vi "set password protection on all VIs.vi"() -> ()   [LabVIEW 2012]
panel:
  in  "keep GFG unlocked":bool
  out "File Path":path
  in  "Confirm New Password":string="password"
  in  "Ring":u16(ring)=2 items=["Unlock", "set new password", "change password"]
  in  "New Password":string="password"
  in  "Old Password":string="password"
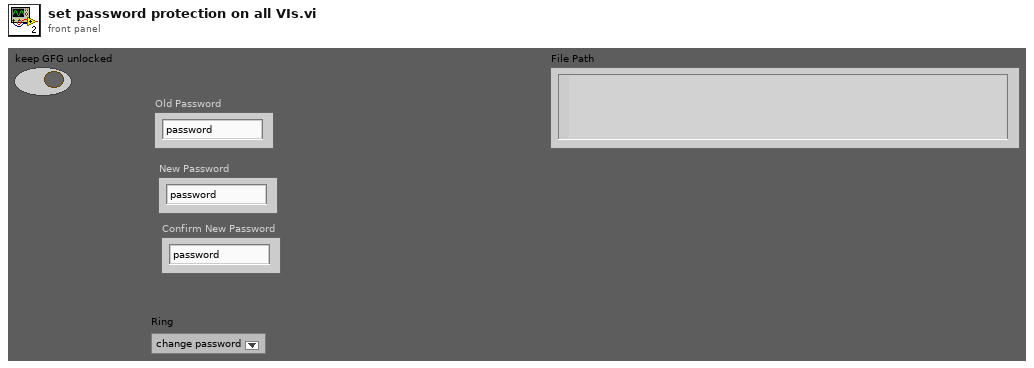
[diagram p1: front panel]
types:
  T1 = enum32{"invalid lock state", "Not Locked", "Locked (No Password)", "Password-protected"}
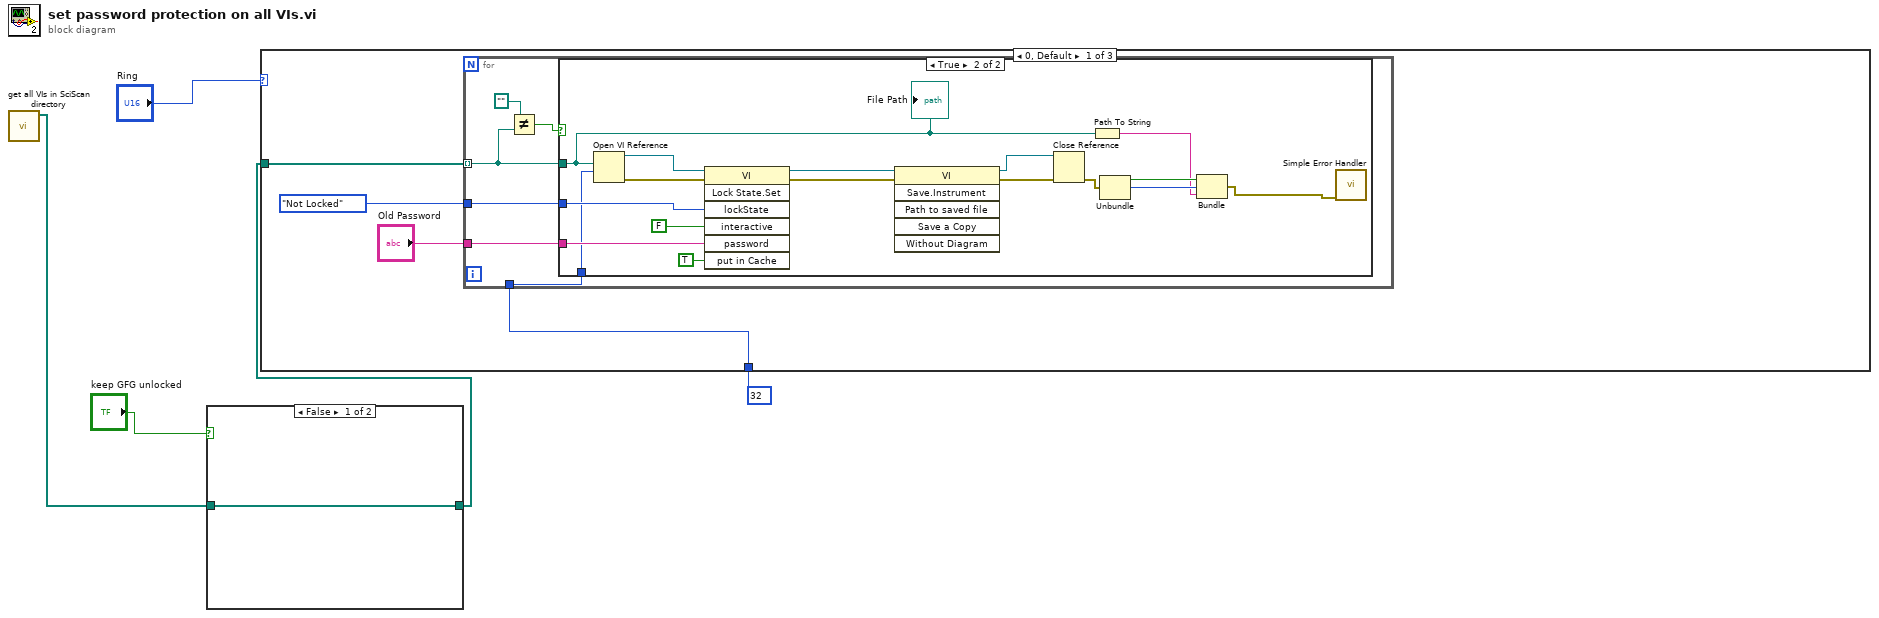
[diagram p0: block diagram]
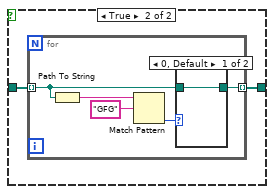
[diagram p2: hidden frame]
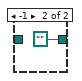
[diagram p3: hidden frame]
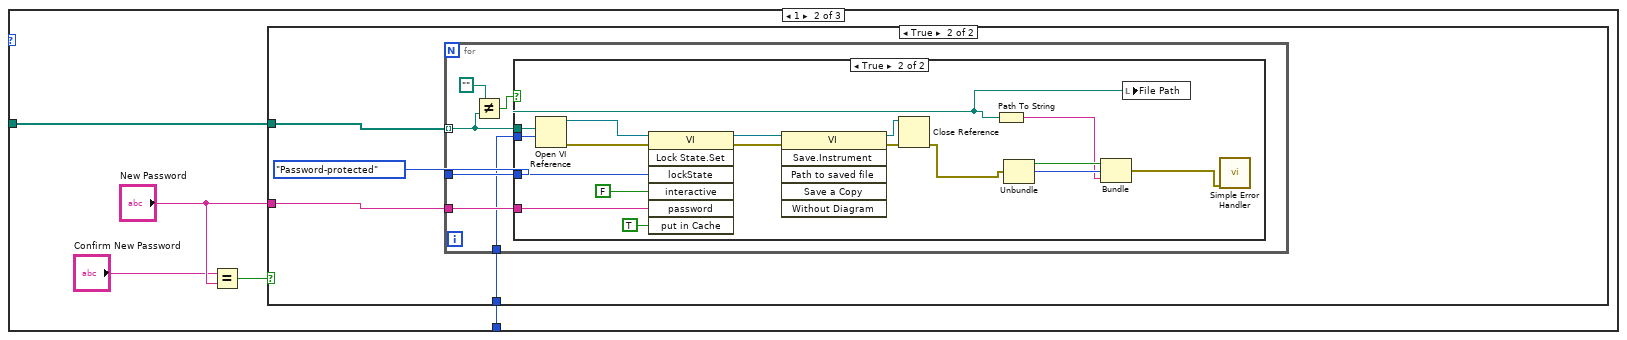
[diagram p5: hidden frame]
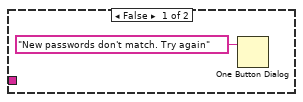
[diagram p6: hidden frame]
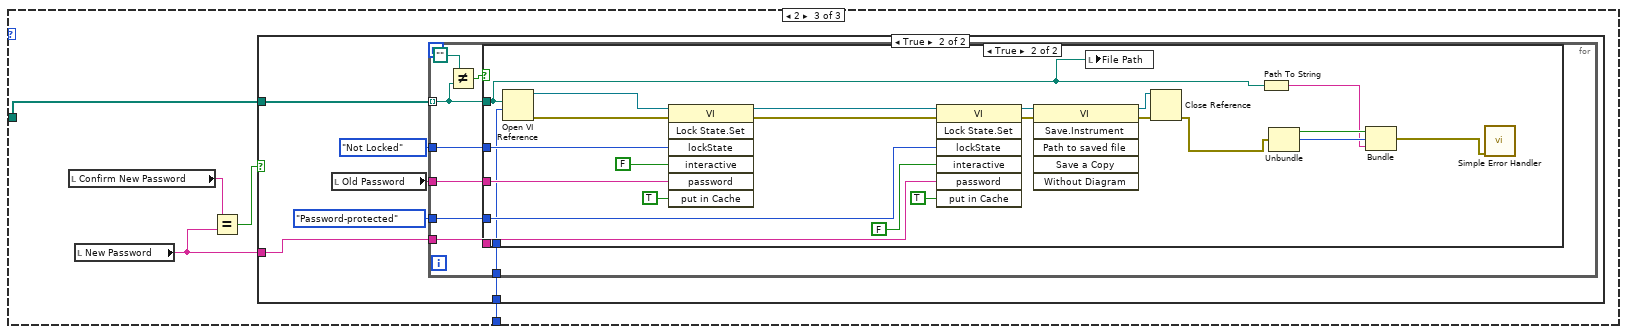
[diagram p8: hidden frame]
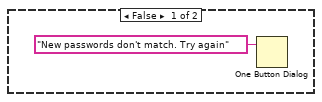
[diagram p9: hidden frame]
diagram:
  n1 = call "get all VIs in SciScan directory.vi"() -> ("All Files in Dir"=w2:path[])  [unwired: 11 in]
  n2 = case shown="False" "keep GFG unlocked" {
    tunnel: [w6 w8] -> w1
    tunnel: w2 -> [w6 w7]
    frame False {
    }
    frame True {
      n3 = for {
        tunnel: [w10] -> w8 mode=indexing
        tunnel: w7 -> [w9] mode=indexing
        n4 = Path To String(path=w9) -> (string=w13:string)
        n5 = Match Pattern(string=w13, regular expression="GFG") -> (offset past match=w11:i32)  [unwired: 1 in, 3 out]
        n6 = case shown="0, Default" w11 {
          tunnel: [w14 path ""] -> w10
          tunnel: w9 -> [w14 _]
          frame 0, Default {
          }
          frame -1 {
          }
        }
      }
    }
  }
  n7 = case shown="0, Default" "Ring" {
    tunnel: w1 -> [w19 w47 w80]
    tunnel: 32 ("options") -> [w16 w43 w76]
    frame 0, Default {
      n8 = for {
        tunnel: w19 -> [w21] mode=indexing
        tunnel: "Old Password" -> [w25]
        tunnel: T1."Not Locked" ("Lock State") -> [w24]
        tunnel: w16 -> [w23]
        n9 = Not Equal?(x=path "", y=w21) -> (x != y?=w20:bool)
        n10 = case shown="True" w20 {
          tunnel: w25 -> [_ w34]
          tunnel: w24 -> [_ w33]
          tunnel: w23 -> [_ w27]
          tunnel: w21 -> [_ w26]
          frame False {
          }
          frame True {
            n11 = Open VI Reference(vi path=w26, options=w27) -> (vi reference=w36:refnum<vi>, error out=w40:errorcluster)  [unwired: 4 in]
            n12 = invoke class="VI" method="Lock State.Set"(reference=w36, error in=w40, "lockState"=w33, "interactive"=FALSE ("Interactive"), "password"=w34, "put in Cache"=TRUE ("Put in Cache")) -> (reference out=w42:refnum<vi>, error out=w41:errorcluster)  [unwired: 1 in, 5 out]
            n13 = invoke class="VI" method="Save.Instrument"(reference=w42, error in=w41) -> (reference out=w37:refnum<vi>, error out=w35:errorcluster)  [unwired: 4 in, 4 out]
            n14 = Close Reference(reference=w37, error in (no error)=w35) -> (error out=w32:errorcluster)
            n15 = Path To String(path=w26) -> (string=w29:string)
            n16 = Unbundle(w32) -> ("status"=w31:bool, "code"=w30:i32)  [unwired: 1 out]
            n17 = Bundle("status"=w31, "code"=w30, w29) -> (w28:cluster{"status":bool, "code":i32, string})  [unwired: 1 in]
            n18 = call <vilib>:"Simple Error Handler.vi"("error in (no error)"=w28) -> ()  [unwired: 4 in, 5 out]
            "File Path" <- w26
          }
        }
      }
    }
    frame 1 {
      n19 = Equal?(x="Confirm New Password", y="New Password") -> (x = y?=w44:bool)
      n20 = case shown="True" w44 {
        tunnel: w47 -> [_ w52]
        tunnel: "New Password" -> [_ w50]
        tunnel: w43 -> [_ w49]
        frame False {
          n21 = One Button Dialog(message="New passwords don't match. Try again") -> ()  [unwired: 1 in, 1 out]
        }
        frame True {
          n22 = for {
            tunnel: w52 -> [w54] mode=indexing
            tunnel: w50 -> [w58]
            tunnel: T1."Password-protected" ("Lock State") -> [w57]
            tunnel: w49 -> [w56]
            n23 = Not Equal?(x=path "", y=w54) -> (x != y?=w53:bool)
            n24 = case shown="True" w53 {
              tunnel: w58 -> [_ w67]
              tunnel: w57 -> [_ w66]
              tunnel: w54 -> [_ w60]
              tunnel: w56 -> [_ w59]
              frame False {
              }
              frame True {
                n25 = Open VI Reference(vi path=w60, options=w59) -> (vi reference=w69:refnum<vi>, error out=w73:errorcluster)  [unwired: 4 in]
                n26 = invoke class="VI" method="Lock State.Set"(reference=w69, error in=w73, "lockState"=w66, "interactive"=FALSE ("Interactive"), "password"=w67, "put in Cache"=TRUE ("Put in Cache")) -> (reference out=w75:refnum<vi>, error out=w74:errorcluster)  [unwired: 1 in, 5 out]
                n27 = invoke class="VI" method="Save.Instrument"(reference=w75, error in=w74) -> (reference out=w70:refnum<vi>, error out=w68:errorcluster)  [unwired: 4 in, 4 out]
                n28 = Close Reference(reference=w70, error in (no error)=w68) -> (error out=w61:errorcluster)
                n29 = Path To String(path=w60) -> (string=w62:string)
                n30 = Unbundle(w61) -> ("status"=w64:bool, "code"=w63:i32)  [unwired: 1 out]
                n31 = Bundle("status"=w64, "code"=w63, w62) -> (w65:cluster{"status":bool, "code":i32, string})  [unwired: 1 in]
                n32 = local write "File Path"(w60) -> ()
                n33 = call <vilib>:"Simple Error Handler.vi"("error in (no error)"=w65) -> ()  [unwired: 4 in, 5 out]
              }
            }
          }
        }
      }
    }
    frame 2 {
      n34 = local read "Confirm New Password"() -> (w79:string)
      n35 = local read "New Password"() -> (w78:string)
      n36 = Equal?(x=w79, y=w78) -> (x = y?=w77:bool)
      n37 = case shown="True" w77 {
        tunnel: w80 -> [_ w87]
        tunnel: w78 -> [_ w84]
        tunnel: w76 -> [_ w82]
        frame False {
          n38 = One Button Dialog(message="New passwords don't match. Try again") -> ()  [unwired: 1 in, 1 out]
        }
        frame True {
          n39 = local read "Old Password"() -> (w85:string)
          n40 = for {
            tunnel: w87 -> [w89] mode=indexing
            tunnel: w85 -> [w95]
            tunnel: T1."Not Locked" ("Lock State") -> [w94]
            tunnel: w84 -> [w93]
            tunnel: T1."Password-protected" ("Lock State") -> [w92]
            tunnel: w82 -> [w91]
            n41 = Not Equal?(x=path "", y=w89) -> (x != y?=w88:bool)
            n42 = case shown="True" w88 {
              tunnel: w95 -> [_ w112]
              tunnel: w94 -> [_ w111]
              tunnel: w93 -> [_ w106]
              tunnel: w92 -> [_ w105]
              tunnel: w91 -> [_ w97]
              tunnel: w89 -> [_ w96]
              frame False {
              }
              frame True {
                n43 = Open VI Reference(vi path=w96, options=w97) -> (vi reference=w114:refnum<vi>, error out=w118:errorcluster)  [unwired: 4 in]
                n44 = invoke class="VI" method="Lock State.Set"(reference=w114, error in=w118, "lockState"=w111, "interactive"=FALSE ("Interactive"), "password"=w112, "put in Cache"=TRUE ("Put in Cache")) -> (reference out=w110:refnum<vi>, error out=w108:errorcluster)  [unwired: 1 in, 5 out]
                n45 = invoke class="VI" method="Lock State.Set"(reference=w110, error in=w108, "lockState"=w105, "interactive"=FALSE ("Interactive"), "password"=w106, "put in Cache"=TRUE ("Put in Cache")) -> (reference out=w109:refnum<vi>, error out=w107:errorcluster)  [unwired: 1 in, 5 out]
                n46 = invoke class="VI" method="Save.Instrument"(reference=w109, error in=w107) -> (reference out=w115:refnum<vi>, error out=w113:errorcluster)  [unwired: 4 in, 4 out]
                n47 = local write "File Path"(w96) -> ()
                n48 = Close Reference(reference=w115, error in (no error)=w113) -> (error out=w98:errorcluster)
                n49 = Path To String(path=w96) -> (string=w99:string)
                n50 = Unbundle(w98) -> ("status"=w101:bool, "code"=w100:i32)  [unwired: 1 out]
                n51 = Bundle("status"=w101, "code"=w100, w99) -> (w102:cluster{"status":bool, "code":i32, string})  [unwired: 1 in]
                n52 = call <vilib>:"Simple Error Handler.vi"("error in (no error)"=w102) -> ()  [unwired: 4 in, 5 out]
              }
            }
          }
        }
      }
    }
  }
